vi "Serialize.vi"(7 "DestinationFolder":path, 8 "error in":errorcluster, 9 "OwningElement in":refnum<k20>, 10 "Document in":refnum<k20>, 11 "StepRun in":refnum<class "StepRun.lvclass">) -> (0 "error out":errorcluster, 1 "OwningElement out":refnum<k20>, 2 "Document out":refnum<k20>, 3 "StepRun out":refnum<class "StepRun.lvclass">)   [LabVIEW 2021, in "ProligentXMLGenerator.lvlib" / "StepRun.lvclass"]
uses:
  StepRun.lvclass
  StepRun.lvclass/StepRun.ctl
  <vilib>/xml/NI_XML.lvlib
  Base/DOMSupport/DOMSupport.lvlib
  Measure/RealMeasure/RealMeasure.lvclass
  Measure/StringMeasure/StringMeasure.lvclass
  Measure/BooleanMeasure/BooleanMeasure.lvclass
  Measure/IntegerMeasure/IntegerMeasure.lvclass
  Measure/DateTimeMeasure/DateTimeMeasure.lvclass
  Model/Characteristic/Characteristic.lvclass
  Model/Document/Document.lvclass
  Failure/FailureReference/FailureReference.lvclass
  Model/CustomData/CustomData.lvclass
  <vilib>/xml/Close Reference(Node).vi
  Measure/Measure/Measure.lvclass
  Base/ExecutionStatus/ExecutionStatus.lvclass
  C:/Projects/proligent-xml-generator-labview/src/ProligentXMLGenerator/Base/Attribute/Attribute.lvclass
  C:/Projects/proligent-xml-generator-labview/src/ProligentXMLGenerator/Base/ExecutionStatus/ExecutionStatus.lvclass
  Base/Guid/Guid.lvclass
  C:/Projects/proligent-xml-generator-labview/src/ProligentXMLGenerator/Base/NonEmptyString/NonEmptyString.lvclass
  C:/Projects/proligent-xml-generator-labview/src/ProligentXMLGenerator/Base/String/String.lvclass
  C:/Projects/proligent-xml-generator-labview/src/ProligentXMLGenerator/Base/Guid/Guid.lvclass
  Base/NonEmptyString_255/NonEmptyString_255.lvclass
  C:/Projects/proligent-xml-generator-labview/src/ProligentXMLGenerator/Base/NonEmptyString_255/NonEmptyString_255.lvclass
  Base/DateTime/DateTime.lvclass
  C:/Projects/proligent-xml-generator-labview/src/ProligentXMLGenerator/Base/DateTime/DateTime.lvclass
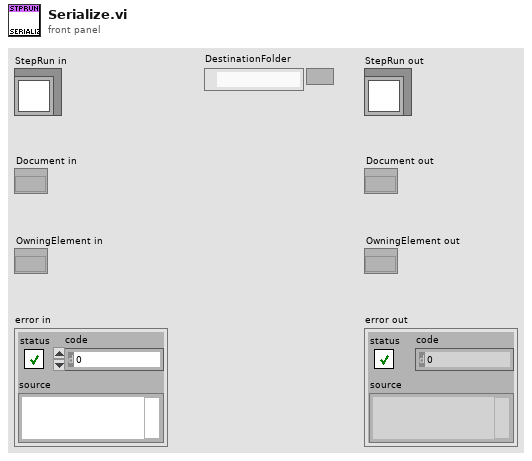
[diagram p1: front panel]
types:
  T1 = typedef "ProligentXMLGenerator.lvlib/StepRun.lvclass/Data.ctl" = cluster{"Name":string, "Measures":refnum<class "Measure.lvclass">[], "FailureReferences":refnum<class "FailureReference.lvclass">[], "Characteristics":refnum<class "Characteristic.lvclass">[], "Documents":refnum<class "Document.lvclass">[], "CustomData":refnum<class "CustomData.lvclass">, "StepExecutionStatus":refnum<class "ExecutionStatus.lvclass">, "StepRunId":refnum<class "Guid.lvclass">, "StepName":refnum<class "NonEmptyString_255.lvclass">, "StartDate":refnum<class "DateTime.lvclass">, "EndDate":refnum<class "DateTime.lvclass">, "TimeZoneInfoId":string}
  T2 = typedef "ProligentXMLGenerator.lvlib/MeasureKind.lvclass/Value.ctl" = enum16{"REAL", "BOOL", "INTEGER", "STRING", "DATETIME"}
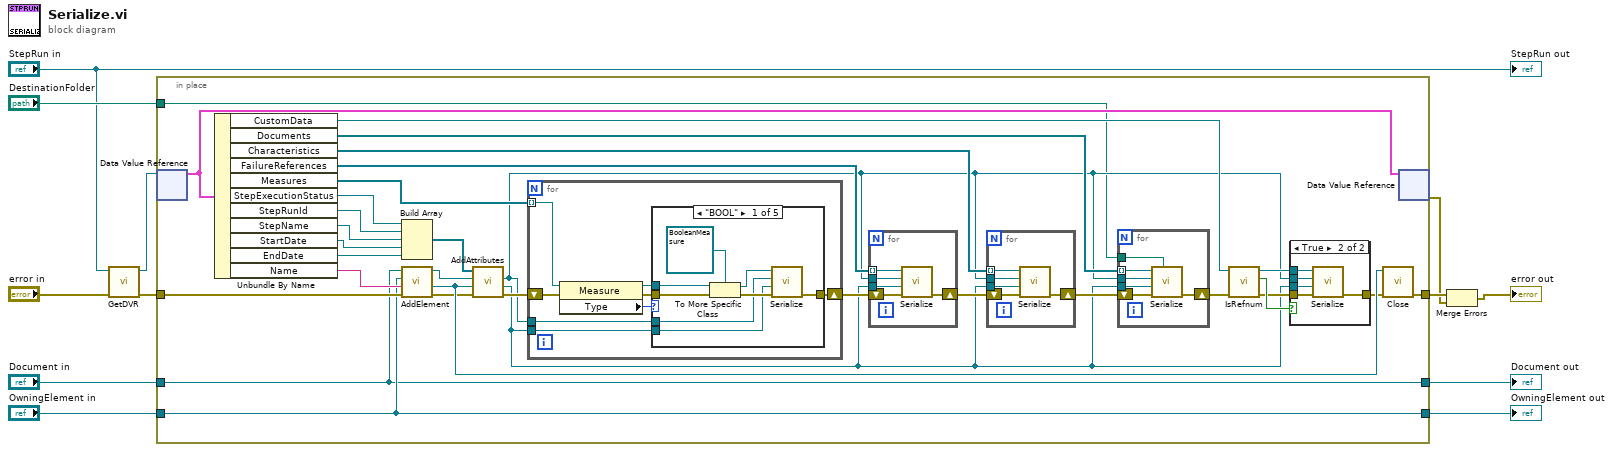
[diagram p0: block diagram]
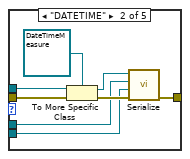
[diagram p2: hidden frame]
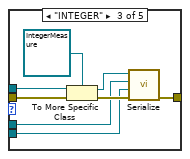
[diagram p3: hidden frame]
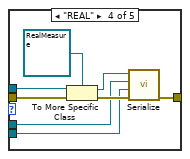
[diagram p4: hidden frame]
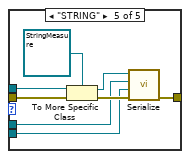
[diagram p5: hidden frame]
diagram:
  n1 = call "GetDVR.vi"("error in"="error in", "StepRun"="StepRun in") -> ("error out"=w5:errorcluster, "DVRReference"=w4:refnum<data-value>)  [unwired: 8 in]
  n2 = in-place "In Place Element Structure" {
    in-place-border: [w44] -> w6
    in-place-border: "Document in" -> [w14]
    in-place-border: w5 -> [w43]
    in-place-border: "OwningElement in" -> [w41]
    in-place-border: [w41] -> w8
    in-place-border: [w14] -> w7
    in-place-border: "DestinationFolder" -> [w13]
    n3 = in-place-dvr #1(w4) -> (w40:T1)  [unwired: 1 out]
    n4 = Unbundle By Name(w40) -> ("CustomData"=w18:refnum<class "CustomData.lvclass">, "Documents"=w19:refnum<class "Document.lvclass">[], "Characteristics"=w20:refnum<class "Characteristic.lvclass">[], "FailureReferences"=w21:refnum<class "FailureReference.lvclass">[], "Measures"=w30:refnum<class "Measure.lvclass">[], "StepExecutionStatus"=w39:refnum<class "ExecutionStatus.lvclass">, "StepRunId"=w22:refnum<class "Guid.lvclass">, "StepName"=w38:refnum<class "NonEmptyString_255.lvclass">, "StartDate"=w37:refnum<class "DateTime.lvclass">, "EndDate"=w36:refnum<class "DateTime.lvclass">, "Name"=w42:string)
    n5 = Build Array(w39, w22, w38, w37, w36) -> (w32:refnum<class "Attribute.lvclass">[])
    n6 = call "AddElement.vi"("error in"=w43, "Name"=w42, "OwningElement in"=w41, "Document in"=w14) -> ("error out"=w33:errorcluster, "NewElement"=w34:refnum<k20>, "Document out"=w35:refnum<k20>)  [unwired: 4 in, 1 out]
    n7 = call "AddAttributes.vi"("error in"=w33, "OwningElement in"=w34, "Document in"=w35, "Attributes"=w32) -> ("error out"=w31:errorcluster, "OwningElement out"=w17:refnum<k20>, "Document out"=w16:refnum<k20>)  [unwired: 5 in]
    n8 = for {
      shift-right: [w49] -> w26
      shift-left: w31 -> [w47]
      tunnel: w30 -> [w48] mode=indexing
      tunnel: w16 -> [w46]
      tunnel: w17 -> [w45]
      n9 = property on="Property Node" class="Measure"(reference=w48, error in=w47) -> (reference out=w51:refnum<class "Measure.lvclass">, error out=w52:errorcluster, "Type"=w50:T2)
      n10 = case shown="\"BOOL\"" w50 {
        tunnel: w52 -> [w60 w68 w76 w84 w92]
        tunnel: w51 -> [w56 w64 w72 w80 w88]
        tunnel: [w58 w66 w74 w82 w90] -> w49
        tunnel: w46 -> [w54 w62 w70 w78 w86]
        tunnel: w45 -> [w53 w61 w69 w77 w85]
        frame "BOOL" {
          n11 = To More Specific Class(target class=refnum<class "BooleanMeasure.lvclass"> refnum ("ProligentResultProcessor:BooleanMeasure"), reference=w56, error in=w60) -> (specific class reference=w55:refnum<class "BooleanMeasure.lvclass">, error out=w59:errorcluster)
          n12 = call "Serialize.vi"("error in"=w59, "OwningElement in"=w53, "Document in"=w54, "BooleanMeasure in"=w55) -> ("error out"=w58:errorcluster)  [unwired: 4 in, 3 out]
        }
        frame "DATETIME" {
          n13 = To More Specific Class(target class=refnum<class "DateTimeMeasure.lvclass"> refnum ("ProligentResultProcessor:DateTimeMeasure"), reference=w64, error in=w68) -> (specific class reference=w63:refnum<class "DateTimeMeasure.lvclass">, error out=w67:errorcluster)
          n14 = call "Serialize.vi"("error in"=w67, "OwningElement in"=w61, "Document in"=w62, "DateTimeMeasure in"=w63) -> ("error out"=w66:errorcluster)  [unwired: 4 in, 3 out]
        }
        frame "INTEGER" {
          n15 = To More Specific Class(target class=refnum<class "IntegerMeasure.lvclass"> refnum ("ProligentResultProcessor:RealMeasure"), reference=w72, error in=w76) -> (specific class reference=w71:refnum<class "IntegerMeasure.lvclass">, error out=w75:errorcluster)
          n16 = call "Serialize.vi"("error in"=w75, "OwningElement in"=w69, "Document in"=w70, "IntergerMeasure in"=w71) -> ("error out"=w74:errorcluster)  [unwired: 4 in, 3 out]
        }
        frame "REAL" {
          n17 = To More Specific Class(target class=refnum<class "RealMeasure.lvclass"> refnum ("ProligentResultProcessor:RealMeasure"), reference=w80, error in=w84) -> (specific class reference=w79:refnum<class "RealMeasure.lvclass">, error out=w83:errorcluster)
          n18 = call "Serialize.vi"("error in"=w83, "OwningElement in"=w77, "Document in"=w78, "RealMeasure in"=w79) -> ("error out"=w82:errorcluster)  [unwired: 4 in, 3 out]
        }
        frame "STRING" {
          n19 = To More Specific Class(target class=refnum<class "StringMeasure.lvclass"> refnum ("ProligentResultProcessor:StringMeasure"), reference=w88, error in=w92) -> (specific class reference=w87:refnum<class "StringMeasure.lvclass">, error out=w91:errorcluster)
          n20 = call "Serialize.vi"("error in"=w91, "OwningElement in"=w85, "Document in"=w86, "StringMeasure in"=w87) -> ("error out"=w90:errorcluster)  [unwired: 4 in, 3 out]
        }
      }
    }
    n21 = for {
      tunnel: w21 -> [w97] mode=indexing
      tunnel: w17 -> [w95]
      tunnel: w16 -> [w96]
      shift-right: [w93] -> w25
      shift-left: w26 -> [w94]
      n22 = call "Serialize.vi"("error in"=w94, "OwningElement in"=w95, "Document in"=w96, "FailureReference in"=w97) -> ("error out"=w93:errorcluster)  [unwired: 4 in, 3 out]
    }
    n23 = for {
      tunnel: w20 -> [w114] mode=indexing
      tunnel: w17 -> [w112]
      tunnel: w16 -> [w113]
      shift-right: [w110] -> w24
      shift-left: w25 -> [w111]
      n24 = call "Serialize.vi"("error in"=w111, "OwningElement in"=w112, "Document in"=w113, "DocumentType in"=w114) -> ("error out"=w110:errorcluster)  [unwired: 4 in, 3 out]
    }
    n25 = for {
      tunnel: w19 -> [w109] mode=indexing
      tunnel: w17 -> [w107]
      tunnel: w16 -> [w108]
      shift-right: [w105] -> w23
      shift-left: w24 -> [w106]
      tunnel: w13 -> [w104]
      n26 = call "Serialize.vi"("DestinationFolder"=w104, "error in"=w106, "OwningElement in"=w107, "Document in"=w108, "DocumentType in"=w109) -> ("error out"=w105:errorcluster)  [unwired: 3 in, 3 out]
    }
    n27 = call "IsRefnum.vi"("error in"=w23, "CustomDataType in"=w18) -> ("error out"=w27:errorcluster, "IsRefnum"=w29:bool, "CustomDataType out"=w28:refnum<class "CustomData.lvclass">)  [unwired: 7 in]
    n28 = case shown="True" w29 {
      tunnel: w16 -> [_ w100]
      tunnel: w27 -> [w98 w103]
      tunnel: [w98 w102] -> w15
      tunnel: w28 -> [_ w101]
      tunnel: w17 -> [_ w99]
      frame False {
      }
      frame True {
        n29 = call "Serialize.vi"("error in"=w103, "OwningElement in"=w99, "Document in"=w100, "CustomDataType in"=w101) -> ("error out"=w102:errorcluster)  [unwired: 4 in, 3 out]
      }
    }
    n30 = call-poly <vilib>:"Close.vi"("error in (no error)"=w15, "node"=w34) -> ("error out"=w44:errorcluster)  [unwired: 7 in]
    n31 = in-place-dvr #1(w40) -> (w3:errorcluster)  [unwired: 1 out]
  }
  "Document out" <- w7
  "OwningElement out" <- w8
  n32 = Merge Errors(w6, w3) -> (→"error out":errorcluster)
  "StepRun out" <- "StepRun in"
